vi "GEN_User Defined Paths.vi"() -> (3 "UserDefinedPath":T1)   [LabVIEW 2016]
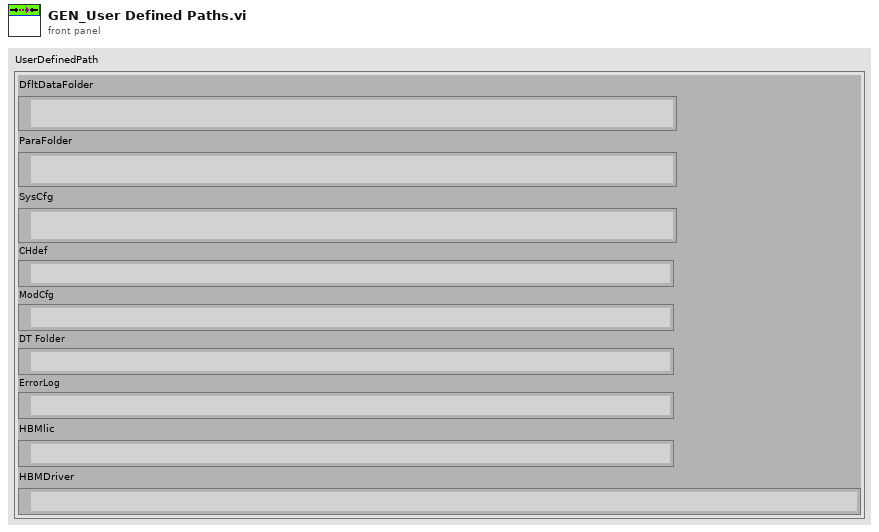
[diagram p1: front panel]
types:
  T1 = cluster{"DfltDataFolder":path, "ParaFolder":path, "SysCfg":path, "CHdef":path, "ModCfg":path, "DT Folder":path, "ErrorLog":path, "HBMlic":path, "HBMDriver":path}
  T2 = enum32{"invalid app kind", "Development System", "Run Time System", "Student Edition", "Embedded LabVIEW", "Evaluation", "Custom"}
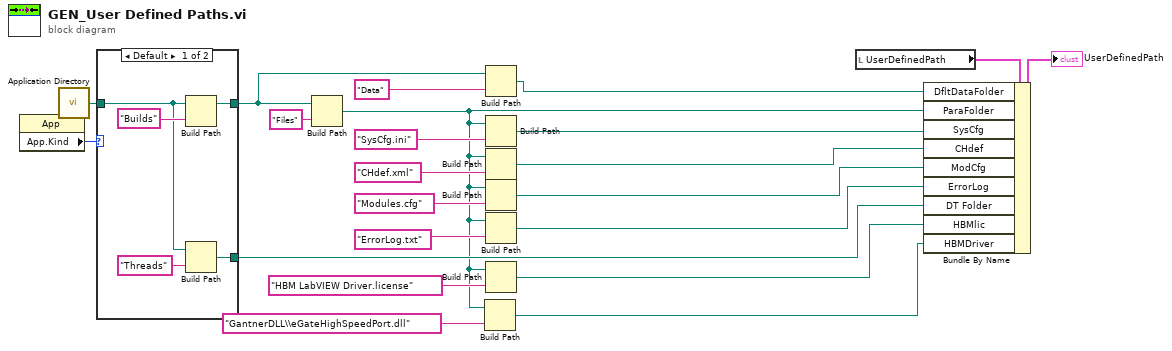
[diagram p0: block diagram]
diagram:
  n1 = property class="App"() -> ("App.Kind"=w19:T2)  [unwired: 2 in, 2 out]
  n2 = call <vilib>:"Application Directory.vi"() -> ("Application Directory"=w22:path)
  n3 = case shown="Default" w19 {
    tunnel: w22 -> [w25 w28]
    tunnel: [w26 w28] -> w6
    tunnel: [w23 w28] -> w14
    frame Default {
      n4 = Build Path(base path=w25, name or relative path="Builds" ("名称或相对路径")) -> (appended path=w26:path)
      n5 = Build Path(base path=w25, name or relative path="Threads" ("名称或相对路径")) -> (appended path=w23:path)
    }
    frame "Run Time System" {
    }
  }
  n6 = Build Path(base path=w6, name or relative path="Files" ("名称或相对路径")) -> (appended path=w1:path)
  n7 = Build Path(base path=w1, name or relative path="GantnerDLL\\eGateHighSpeedPort.dll" ("名称或相对路径")) -> (appended path=w2:path)
  n8 = Build Path(base path=w6, name or relative path="Data" ("名称或相对路径")) -> (appended path=w4:path)
  n9 = Build Path(base path=w1, name or relative path="SysCfg.ini" ("名称或相对路径")) -> (appended path=w16:path)
  n10 = Build Path(base path=w1, name or relative path="CHdef.xml" ("名称或相对路径")) -> (appended path=w15:path)
  n11 = Build Path(base path=w1, name or relative path="Modules.cfg" ("名称或相对路径")) -> (appended path=w12:path)
  n12 = Build Path(base path=w1, name or relative path="ErrorLog.txt" ("名称或相对路径")) -> (appended path=w9:path)
  n13 = Build Path(base path=w1, name or relative path="HBM LabVIEW Driver.license" ("名称或相对路径")) -> (appended path=w7:path)
  n14 = local read "UserDefinedPath"() -> (w21:T1)
  n15 = Bundle By Name(cluster=w21, "DfltDataFolder"=w4, "ParaFolder"=w1, "SysCfg"=w16, "CHdef"=w15, "ModCfg"=w12, "ErrorLog"=w9, "DT Folder"=w14, "HBMlic"=w7, "HBMDriver"=w2) -> (→"UserDefinedPath":T1)
